vi "Get All Project VI Data.vi"(8 "error in":errorcluster, 11 "Lvproj Path":path) -> (0 "error out":errorcluster, 3 "Item Data":refnum<class "Item.lvclass">[](array[class]))   [LabVIEW 2020, in "VI Properties Editor.lvlib"]
doc: "Gets all VI data from a project located at <B>Path</B>."
uses:
  VI Properties Editor.lvlib
  <vilib>/xml/NI_XML.lvlib
  <vilib>/xml/Close Reference(Node).vi
  CTLs/XPath Get Attribute.ctl
  Classes/Item/Item.lvclass
  <vilib>/xml/Load XML String.vi
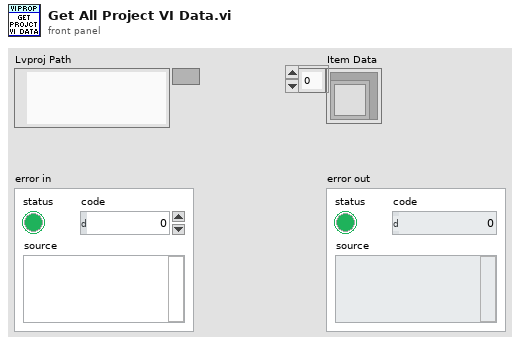
[diagram p1: front panel]
types:
  T1 = typedef "VI Properties Editor.lvlib/XPath Get Attribute.ctl" = enum16{"Item[@Type='VI']/@URL", "Item[@Type='LVClass']/@URL", "Item[@Type='Library']/@URL", "Item[@Type='Folder' and not (@URL)]/@Name", "@Name"}
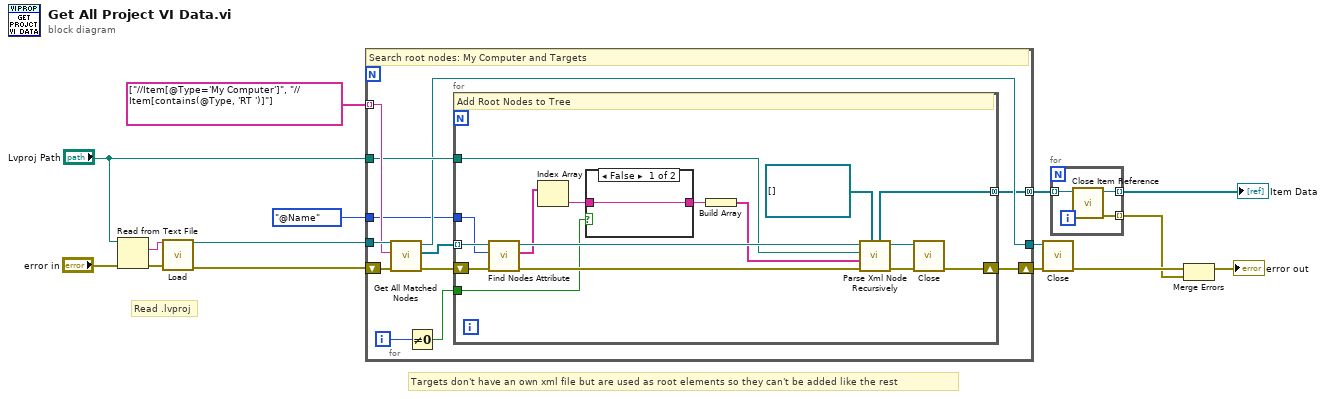
[diagram p0: block diagram]
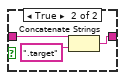
[diagram p2: hidden frame]
diagram:
  # "Targets don't have an own xml file but are used as root elements so they can't be added like the rest"
  # "Read .lvproj"
  n1 = Read from Text File(file (use dialog)="Lvproj Path", error in="error in") -> (text=w14:string, error out=w13:errorcluster)  [unwired: 2 in, 2 out]
  n2 = call-poly <vilib>:"Load.vi"("XML string"=w14, "error in (no error)"=w13) -> ("DOM document out"=w15:refnum<k20>, "error out"=w11:errorcluster)  [unwired: 11 in, 1 out]
  n3 = for {
    tunnel: w15 -> [w27]
    tunnel: string[] ["//Item[@Type='My Computer']", "//Item[contains(@Type, 'RT ')]"] -> [w26] mode=indexing
    tunnel: "Lvproj Path" -> [w25]
    shift-right: [w24] -> w12
    shift-left: w11 -> [w22]
    tunnel: [w20] -> w9
    tunnel: XPath_Get_Attribute."@Name" ("XPath") -> [w19]
    tunnel: [w18] -> w2 mode=concatenating
    i -> [w16]
    # "Search root nodes: My Computer and Targets"
    n4 = call <vilib>:"Get All Matched Nodes.vi"("error in (no error)"=w22, "XPath expression"=w26, "node in"=w27) -> ("error out"=w21:errorcluster, "node result array"=w23:refnum<k20>[], "node out"=w20:refnum<k20>)  [unwired: 6 in]
    n5 = Not Equal To 0?(x=w16) -> (x != 0?=w17:bool)
    n6 = for {
      tunnel: w25 -> [w34]
      tunnel: w23 -> [w43] mode=indexing
      shift-right: [w40] -> w24
      shift-left: w21 -> [w39]
      tunnel: w19 -> [w37]
      tunnel: [w30] -> w18 mode=concatenating
      tunnel: w17 -> [w29]
      # "Add Root Nodes to Tree"
      n7 = call "Find Nodes Attribute.vi"("error in (no error)"=w39, "XPath"=w37, "Node in"=w43) -> ("error out"=w38:errorcluster, "Attribute"=w33:string[], "Node out"=w42:refnum<k20>)  [unwired: 6 in]
      n8 = Index Array(array=w33) -> (element=w36:string)  [unwired: 1 in]
      n9 = case shown="False" w29 {
        tunnel: w36 -> [w44 w47]
        tunnel: [w44 w46] -> w35
        frame False {
        }
        frame True {
          n10 = Concatenate Strings(w47, ".target" ("string")) -> (w46:string)
        }
      }
      n11 = Build Array(w35) -> (w32:string[])
      n12 = call "Parse Xml Node Recursively.vi"("Item Data"=refnum<class "Item.lvclass">[] [], "error in"=w38, "Parents"=w32, "XML File Path"=w34, "Node in"=w42) -> ("error out"=w41:errorcluster, "Node out"=w31:refnum<k20>, "Item Data out"=w30:refnum<class "Item.lvclass">[])  [unwired: 4 in]
      n13 = call-poly <vilib>:"Close.vi"("error in (no error)"=w41, "node"=w31) -> ("error out"=w40:errorcluster)  [unwired: 7 in]
    }
  }
  n14 = call-poly <vilib>:"Close.vi"("error in (no error)"=w12, "node"=w9) -> ("error out"=w5:errorcluster)  [unwired: 7 in]
  n15 = for {
    tunnel: [w50] -> w4 mode=indexing
    tunnel: w2 -> [w49] mode=indexing
    tunnel: [w48] -> w1 mode=indexing
    n16 = call-dynamic "Close Item Reference.vi"("Item in"=w49) -> ("error out"=w50:errorcluster, "Item out"=w48:refnum<class "Item.lvclass">)  [unwired: 9 in]
  }
  "Item Data" <- w1
  n17 = Merge Errors(w5, w4) -> (→"error out":errorcluster)
